vi "Initialize.vi"(7 "baud rate (9600)":u32=9600, 8 "error In":errorcluster, 9 "Query Instrument":bool, 10 "parity (0:none)":enum16{"None", "Odd", "Even", "Mark", "Space"}(ring), 11 "VISA resource name":refnum<visa-resource-name>) -> (0 "error out":errorcluster, 2 "read buffer":string="\r\n", 3 "VISA resource name out":refnum<visa-resource-name>)   [LabVIEW 2013, in "Fluke 2625A.lvlib"]
doc: "Establishes communication with the instrument and optionally performs an instrument identification query and/or an instrument reset. It also places the instrument in a default state needed for other instrument driver operations. Therefore, call this VI before calling other instrument driver VIs for this instrument. Generally, you need to call the Initialize VI only once at the beginning of an application."
uses:
  <instrlib>/Fluke 2625A/Fluke 2625A.lvlib
  <vilib>/Instr/_visa.llb/VISA Open Access Mode.ctl
  <vilib>/Instr/_visa.llb/VISA Configure Serial Port (Instr).vi
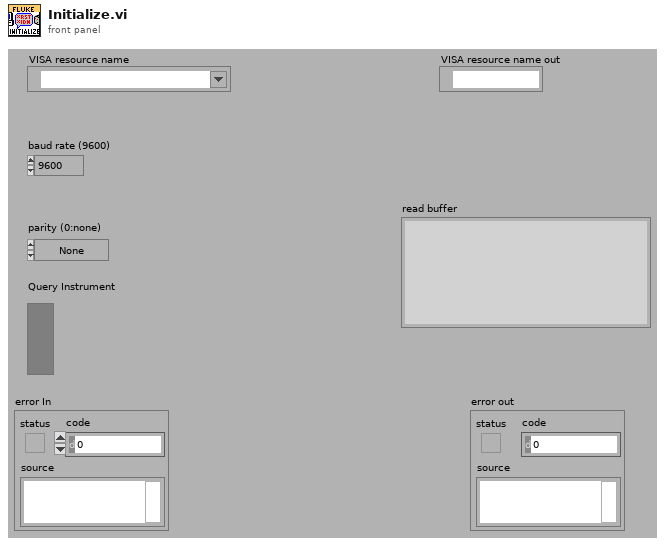
[diagram p1: front panel]
types:
  T1 = typedef "VISA Open Access Mode.ctl" = u32
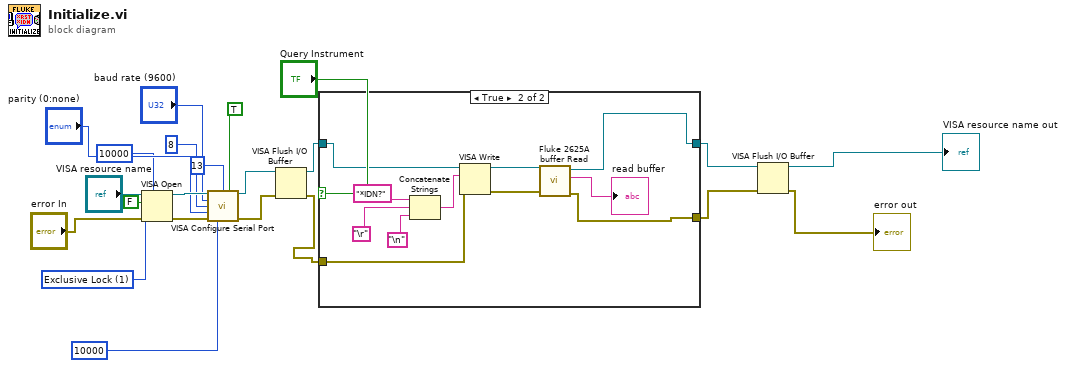
[diagram p0: block diagram]
diagram:
  w2 = T1 1 items=["VISA Defaults"=0, "Exclusive Lock"=1, "Load Configured Settings"=4] ("Access Mode")
  n1 = VISA Open(timeout (0)=u32 10000 ("VISA Open timeout (0)"), duplicate session (F)=FALSE, access mode=w2, error in (no error)="error In", VISA resource name="VISA resource name") -> (VISA resource name=w21:refnum<visa-resource-name>, error out=w20:errorcluster)
  n2 = call-poly "VISA Configure Serial Port"("VISA resource name"=w21, "timeout (10sec)"=u32 10000, "termination char\n(0xA = '\\n' = LF)"=u8 13 ("termination char\n(0xA = '\\n' = LF)"), "Enable Termination\nChar (T)"=TRUE ("Enable Termination\nChar (T)"), "baud rate (9600)"="baud rate (9600)", "data bits (8)"=u16 8, "parity (0:none)"="parity (0:none)", "error in (no error)"=w20) -> ("VISA resource name out"=w7:refnum<visa-resource-name>, "error out"=w6:errorcluster)  [unwired: 6 in]
  n3 = VISA Flush I/O Buffer(VISA resource name=w7, error in (no error)=w6) -> (VISA resource name out=w8:refnum<visa-resource-name>, error out=w9:errorcluster)  [unwired: 1 in]
  n4 = case shown="True" "Query Instrument" {
    tunnel: w8 -> [w23 w33]
    tunnel: w9 -> [w24 w31]
    tunnel: [w24 w28] -> w12
    tunnel: [w23 w27] -> w13
    frame False {
    }
    frame True {
      n5 = Concatenate Strings("*IDN?", "\r", "\n") -> (w32:string)
      n6 = VISA Write(VISA resource name=w33, write buffer=w32, error in (no error)=w31) -> (VISA resource name out=w30:refnum<visa-resource-name>, error out=w29:errorcluster)  [unwired: 1 out]
      n7 = call <instrlib>:"Fluke 2625A buffer Read.vi"("error out"=w29, "VISA resource name out"=w30) -> ("error out 2"=w28:errorcluster, "read buffer"=→"read buffer":string, "VISA resource name out 2"=w27:refnum<visa-resource-name>)  [unwired: 7 in]
    }
  }
  n8 = VISA Flush I/O Buffer(VISA resource name=w13, error in (no error)=w12) -> (VISA resource name out=→"VISA resource name out":refnum<visa-resource-name>, error out=→"error out":errorcluster)  [unwired: 1 in]
